vi "deploy default.vi"(10 "data":T1, 11 "in":bool) -> (3 "deploy":bool)   [LabVIEW 2015]
uses:
  eash data.ctl
  USB Template (LV 8.6)/Car Wash/Controls/Wash Options.ctl
  times.ctl
  USB Template (LV 8.6)/Car Wash/Controls/Car Wash Indicators.ctl
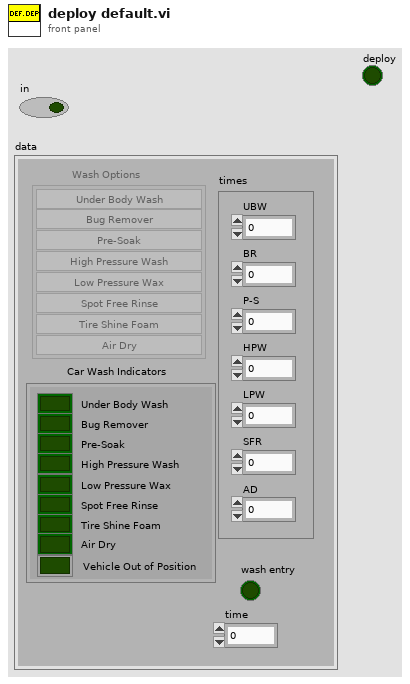
[diagram p1: front panel]
types:
  T1 = typedef "eash data.ctl" = cluster{"Wash Options":T2, "times":T3, "Car Wash Indicators":T4, "wash entry":bool, "time ":dbl}
  T2 = typedef "Wash Options.ctl" = cluster{"Underbody Wash":bool, "Bug Remover":bool, "Pre-Soak":bool, "High Pressure Wash":bool, "Low Pressure Wax":bool, "Spot Free Rinse":bool, "Tire Shine Foam":bool, "Air Dry":bool}
  T3 = typedef "times.ctl" = cluster{"UBW":dbl, "BR":dbl, "P-S":dbl, "HPW":dbl, "LPW":dbl, "SFR":dbl, "AD":dbl}
  T4 = typedef "Car Wash Indicators.ctl" = cluster{"Under Body Wash":bool, "Bug Remover":bool, "Pre-Soak":bool, "High Pressure Wash":bool, "Low Pressure Wax":bool, "Spot Free Rinse":bool, "Tire Shine Foam":bool, "Air Dry":bool, "Vehicle Out of Position":bool}
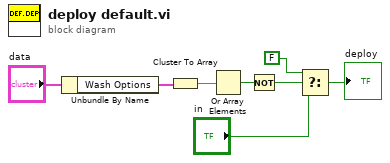
[diagram p0: block diagram]
diagram:
  n1 = Unbundle By Name("data") -> ("Wash Options"=w3:T2)
  n2 = Cluster To Array(cluster=w3) -> (array=w4:bool[])
  n3 = Or Array Elements(Boolean array=w4) -> (logical OR=w5:bool)
  n4 = Not(x=w5) -> (.not. x?=w6:bool)
  n5 = Select(t=FALSE, s=w6, f="in") -> (s? t:f=→"deploy":bool)
